vi "Timebase_RANFe.vi"(7 "Write?":bool, 8 "Error":errorcluster caption="错误输入（无错误）", 10 "Time(s/div)":dbl, 11 "VISA resource name":refnum<visa-resource-name>) -> (0 "Error out":errorcluster, 2 "Time out(s/div)":dbl, 3 "VISA resource name out":refnum<visa-resource-name>)   [LabVIEW 2020]
doc: "满量程时间"
panel:
  out "读取缓冲区":string
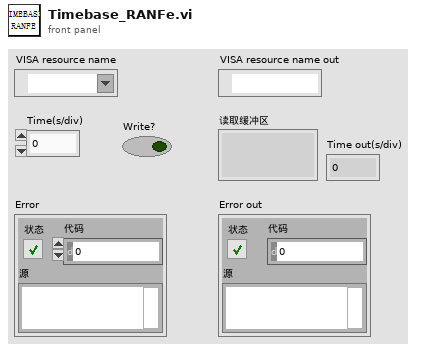
[diagram p1: front panel]
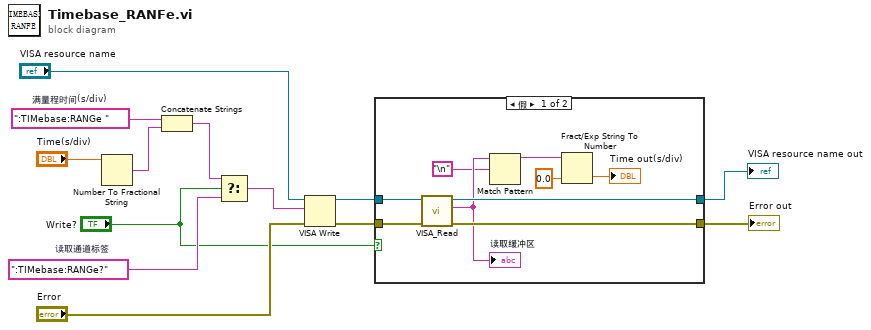
[diagram p0: block diagram]
diagram:
  w8 = ":TIMebase:RANGe?"  # 读取通道标签
  w12 = ":TIMebase:RANGe "  # 满量程时间(s/div)
  n1 = Number To Fractional String(number="Time(s/div)") -> (F-format string=w11:string)  [unwired: 3 in]
  n2 = Concatenate Strings(w12, w11) -> (w9:string)
  n3 = Select(t=w9, s="Write?", f=w8) -> (s? t:f=w7:string)
  n4 = VISA Write(VISA resource name="VISA resource name", write buffer=w7, error in (no error)="Error") -> (VISA resource name out=w3:refnum<visa-resource-name>, error out=w5:errorcluster)  [unwired: 1 out]
  n5 = case shown="假" "Write?" {
    tunnel: w3 -> [w22 w24]
    tunnel: w5 -> [w21 w23]
    tunnel: [w19 w23] -> w4
    tunnel: [w20 w24] -> w1
    frame False {
      n6 = call "VISA_Read.vi"("Error"=w21, "VISA resource name"=w22) -> ("Error out"=w19:errorcluster, "读取缓冲区"=w18:string, "VISA resource name out"=w20:refnum<visa-resource-name>)  [unwired: 7 in]
      "读取缓冲区" <- w18
      n7 = Match Pattern(string=w18, regular expression="\n") -> (before substring=w15:string)  [unwired: 1 in, 3 out]
      n8 = Fract/Exp String To Number(string=w15, default (0 dbl)=0.0 ("默认(0 I32)")) -> (number=→"Time out(s/div)":dbl)  [unwired: 2 in, 1 out]
    }
    frame True {
    }
  }
  "VISA resource name out" <- w1
  "Error out" <- w4
